vi "aggregator - ii.vi"(5 "requested averaging interval":i32=10, 6 "first time":bool, 7 "requested size":i32=20, 11 "number":cdb) -> (0 "interpolated average":cdb, 1 "mean array":cdb[](array[numeric]), 2 "interp array":cdb[](array[numeric]), 3 "Array":cdb[](array[numeric]), 4 "slope":cdb)   [LabVIEW 2015]
panel:
  out "subarray":cdb[](array[numeric])
  out "# of elem":i32
  out "actual number of elements":i32
  out "mean":cdb
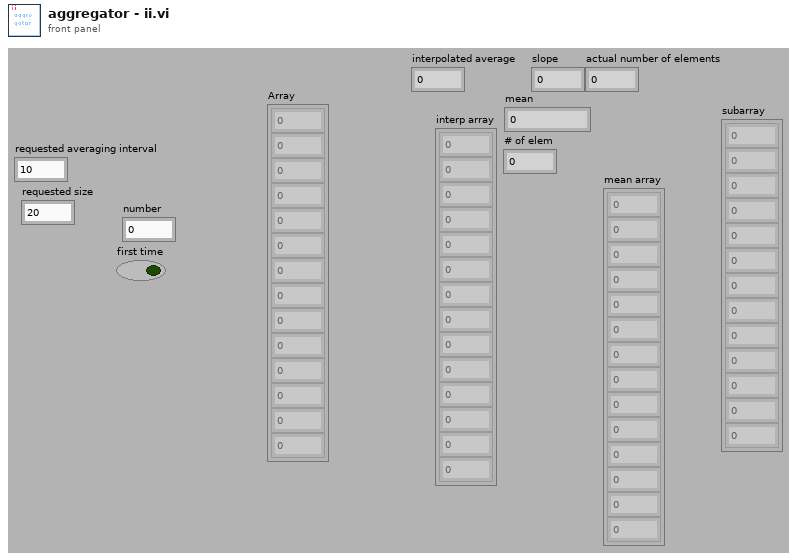
[diagram p1: front panel]
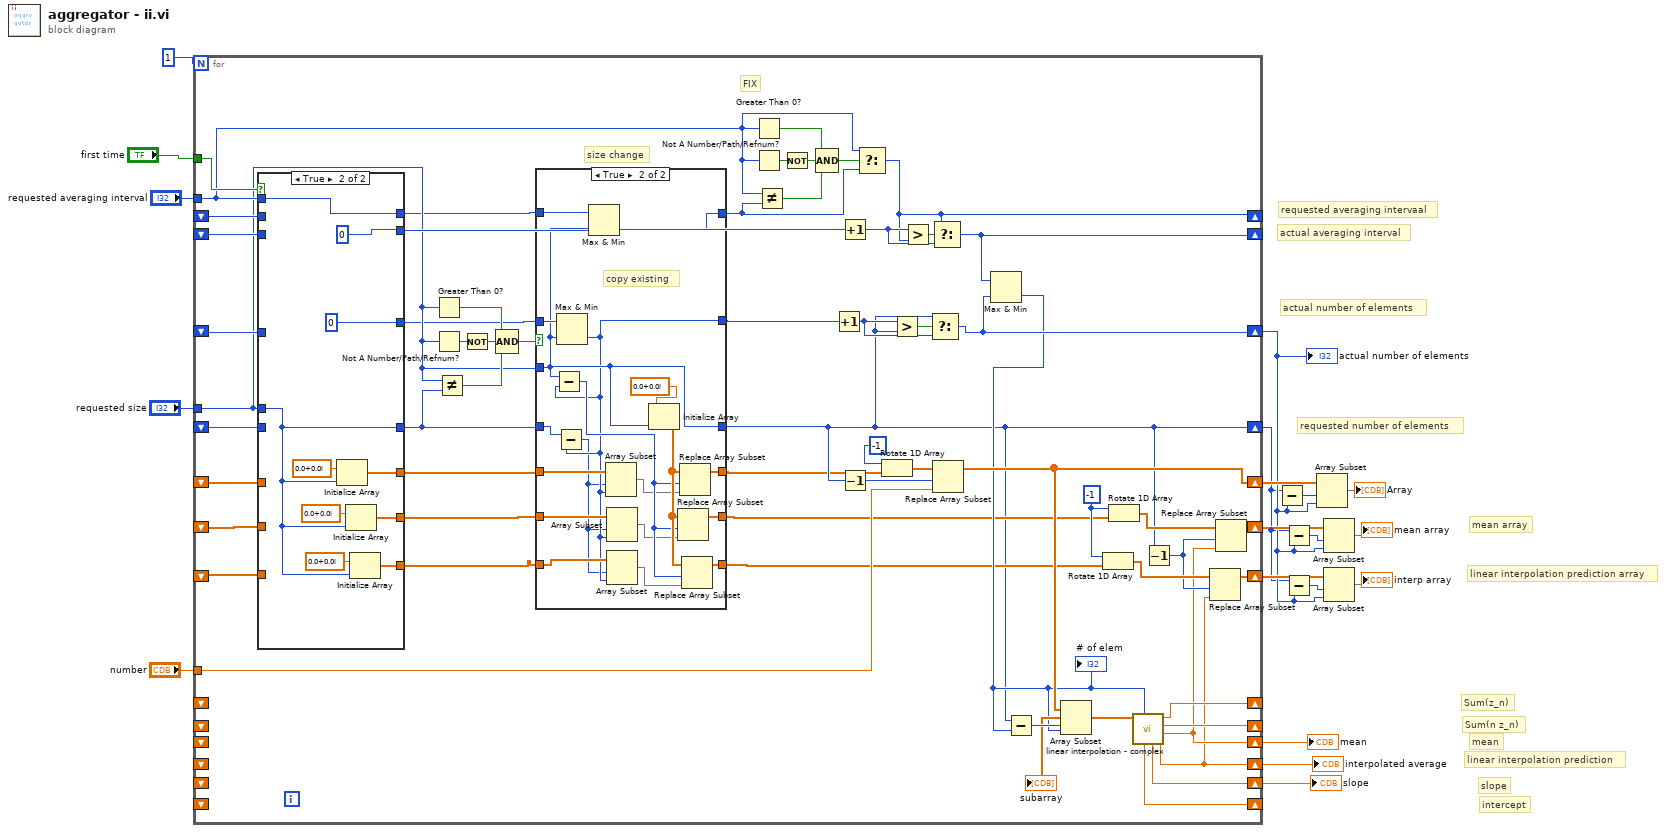
[diagram p0: block diagram]
diagram:
  # "actual averaging interval"
  # "requested averaging intervaal"
  # "linear interpolation prediction"
  # "mean"
  # "intercept"
  # "slope"
  # "linear interpolation prediction array"
  # "mean array"
  # "Sum(n z_n)"
  # "Sum(z_n)"
  # "requested number of elements"
  # "actual number of elements"
  n1 = for {
    N: 1 -> [_]
    tunnel: "first time" -> [w55]
    shift-right: [w36] -> w5
    shift-left: _ -> [w79]
    tunnel: "requested size" -> [w29]
    tunnel: "number" -> [w74]
    shift-right: [w57] -> w15
    shift-left: _ -> [w76]
    shift-right: [w31] -> w4
    shift-left: _ -> [w71]
    shift-right: [w64] -> w9
    shift-left: _ -> [w70]
    shift-right: [w63] -> w6
    shift-left: _ -> [w69]
    shift-right: [w53] -> _
    shift-left: _ -> [_]
    shift-right: [w52] -> _
    shift-left: _ -> [_]
    shift-right: [w49] -> w2
    shift-left: _ -> [_]
    shift-right: [w48] -> _
    shift-left: _ -> [_]
    shift-right: [w51] -> w1
    shift-left: _ -> [_]
    shift-right: [w50] -> w3
    shift-left: _ -> [_]
    shift-right: [w35] -> _
    shift-left: _ -> [w59]
    shift-right: [w37] -> _
    shift-left: _ -> [w58]
    tunnel: "requested averaging interval" -> [w38]
    w66 = -1 ("n")
    # "FIX"
    # "size change"
    n2 = case shown="True" w55 {
      tunnel: w79 -> [w110 _]
      tunnel: [w110 0] -> w28
      tunnel: w76 -> [w107 _]
      tunnel: w29 -> [_ w112]
      tunnel: w71 -> [w108 _]
      tunnel: w70 -> [w106 _]
      tunnel: w69 -> [w105 _]
      tunnel: [w107 w115] -> w24
      tunnel: [w106 w114] -> w25
      tunnel: [w105 w113] -> w23
      tunnel: [w111 0] -> w61
      tunnel: w59 -> [w111 _]
      tunnel: w38 -> [_ w116]
      tunnel: w58 -> [w109 _]
      tunnel: [w109 w116] -> w27
      tunnel: [w108 w112] -> w30
      frame False {
      }
      frame True {
        n3 = Initialize Array(cdb 0.0+0.0i, w112) -> (w115:cdb[])
        n4 = Initialize Array(cdb 0.0+0.0i, w112) -> (w114:cdb[])
        n5 = Initialize Array(cdb 0.0+0.0i, w112) -> (w113:cdb[])
      }
    }
    n6 = Greater Than 0?(x=w29) -> (x > 0?=w46:bool)
    n7 = Not A Number/Path/Refnum?(number/path/refnum=w29) -> (NaN/Path/Refnum?=w47:bool)
    n8 = Not Equal?(x=w29, y=w30) -> (x != y?=w44:bool)
    n9 = Not(x=w47) -> (.not. x?=w45:bool)
    n10 = Compound Arithmetic op=AND(w46, w45, w44) -> (w20:bool)
    n11 = case shown="True" w20 {
      tunnel: [w85 w87] -> w21
      tunnel: w28 -> [w85 w103]
      tunnel: [w84 w95] -> w31
      tunnel: w30 -> [w84 w88]
      tunnel: [w83 w102] -> w22
      tunnel: w24 -> [w83 w94]
      tunnel: w29 -> [_ w95]
      tunnel: w23 -> [w81 w92]
      tunnel: w25 -> [w82 w90]
      tunnel: [w82 w101] -> w33
      tunnel: [w81 w100] -> w32
      tunnel: w27 -> [w80 w97]
      tunnel: [w80 w96] -> w26
      frame False {
      }
      frame True {
        # "copy existing"
        n12 = Max & Min(x=w103, y=w95) -> (min(x,y)=w87:i32)  [unwired: 1 out]
        n13 = Subtract(x=w95, y=w87) -> (x-y=w98:i32)
        n14 = Subtract(x=w88, y=w87) -> (x-y=w86:i32)
        n15 = Max & Min(x=w97, y=w95) -> (min(x,y)=w96:i32)  [unwired: 1 out]
        n16 = Array Subset(array=w94, index=w86, length=w87) -> (w93:cdb[])
        n17 = Array Subset(array=w90, index=w86, length=w87) -> (w89:cdb[])
        n18 = Array Subset(array=w92, index=w86, length=w87) -> (w91:cdb[])
        n19 = Initialize Array(cdb 0.0+0.0i, w95) -> (w99:cdb[])
        n20 = Replace Array Subset(array=w99, new element=w89, index=w98) -> (w101:cdb[])
        n21 = Replace Array Subset(array=w99, new element=w93, index=w98) -> (w102:cdb[])
        n22 = Replace Array Subset(array=w99, new element=w91, index=w98) -> (w100:cdb[])
      }
    }
    n23 = Greater Than 0?(x=w38) -> (x > 0?=w42:bool)
    n24 = Not A Number/Path/Refnum?(number/path/refnum=w38) -> (NaN/Path/Refnum?=w43:bool)
    n25 = Not Equal?(x=w38, y=w26) -> (x != y?=w40:bool)
    n26 = Not(x=w43) -> (.not. x?=w41:bool)
    n27 = Compound Arithmetic op=AND(w42, w41, w40) -> (w39:bool)
    n28 = Increment(x=w21) -> (x+1=w77:i32)
    n29 = Increment(x=w61) -> (x+1=w60:i32)
    n30 = Decrement(x=w31) -> (x-1=w73:i32)
    n31 = Select(t=w38, s=w39, f=w26) -> (s? t:f=w37:i32)
    n32 = Rotate 1D Array(1:w22, 2:-1 ("n")) -> (0:w72:cdb[])
    n33 = Greater?(x=w77, y=w31) -> (0:w78:bool)
    n34 = Greater?(x=w60, y=w37) -> (0:w62:bool)
    n35 = Select(t=w31, s=w78, f=w77) -> (s? t:f=w36:i32)
    n36 = Select(t=w37, s=w62, f=w60) -> (s? t:f=w35:i32)
    n37 = Replace Array Subset(array=w72, new element=w74, index=w73) -> (w57:cdb[])
    n38 = Max & Min(x=w35, y=w36) -> (min(x,y)=w34:i32)  [unwired: 1 out]
    "# of elem" <- w34
    n39 = Subtract(x=w31, y=w34) -> (x-y=w56:i32)
    n40 = Array Subset(array=w57, index=w56, length=w34) -> (w54:cdb[])
    "subarray" <- w54
    n41 = Rotate 1D Array(1:w32, 2:w66) -> (0:w67:cdb[])
    n42 = Rotate 1D Array(1:w33, 2:w66) -> (0:w68:cdb[])
    n43 = call "linear interpolation - complex.vi"("n"=w34, "Array"=w54) -> ("interpolated average"=w50:cdb, "mean"=w51:cdb, "sum n z_n"=w52:cdb, "sum z_n"=w53:cdb, "slope"=w49:cdb, "intercept"=w48:cdb)  [unwired: 3 in, 1 out]
    n44 = Decrement(x=w31) -> (x-1=w65:i32)
    n45 = Replace Array Subset(array=w67, new element=w50, index=w65) -> (w63:cdb[])
    n46 = Replace Array Subset(array=w68, new element=w51, index=w65) -> (w64:cdb[])
  }
  "interpolated average" <- w3
  "slope" <- w2
  "mean" <- w1
  "actual number of elements" <- w5
  n47 = Subtract(x=w4, y=w5) -> (x-y=w13:i32)
  n48 = Subtract(x=w4, y=w5) -> (x-y=w10:i32)
  n49 = Subtract(x=w4, y=w5) -> (x-y=w7:i32)
  n50 = Array Subset(array=w15, index=w13, length=w5) -> (→"Array":cdb[])
  n51 = Array Subset(array=w9, index=w10, length=w5) -> (→"mean array":cdb[])
  n52 = Array Subset(array=w6, index=w7, length=w5) -> (→"interp array":cdb[])
